vi "Serial_W_R with Files.vi"() -> ()   [LabVIEW 2022 SP3]
doc: "This example performs writes and reads on a serial port, as directed by the user. You can press the Write and Read buttons, and change the Read Count, while the example is running.\n\nThe parameters set for the serial port must match the parameters of the connected instrument or device. In this example, the Read Count parameter specifies the number of bytes that the serial port reads. If there were more bytes at the port than the specified number, those bytes would not be read. If there were less bytes at the port than the specified number, you would receive a timeout error.\n\nThis example expands upon the flow control options for XON and XOFF, allowing the user to choose those control characters. Also, the user can enable or disable a termination character. Some devices require a termination character in order to identify the end of command strings. Some devices send a termination character to signify the end of data to be read. This example shows how you can end the Read operation once a termination character is detected in the buffer and/or append a termination character at the end of the Write data."
uses:
  Applications/National Instruments/LabVIEW 2022 64-bit/examples/Instrument IO/Serial/support/Serial - Settings.ctl
  Applications/National Instruments/LabVIEW 2022 64-bit/examples/Instrument IO/Serial/support/Serial - ASCII Characters.ctl
  Applications/National Instruments/LabVIEW 2022 64-bit/examples/Instrument IO/Serial/support/Serial - XON-XOFF Characters.ctl
  Command_buttons.ctl
  <vilib>/Instr/_visa.llb/VISA Configure Serial Port (Instr).vi
  fg_enum.ctl
panel:
  in  "Stop Tx":bool
  in  "Temperature\nto set":dbl
  in  "Command Radio\nButtons":T1
  out "Response":string
  in  "Write":bool
  in  "Read":bool
  in  "VISA resource name":refnum<visa-resource-name>="COM1"
  # "------------------------\nPROGRAM EXECUTION   \n------------------------\n1. Connect PolyStat controller to PC via RS232 cable and choose corresponding port in 'VISA resource name'\n2. Set the time to poll which decides the time interval between each write-read pair or how often the command must be written and read\n3. Choose command to run by clicking the Radio buttons (can be changed during run). Refer the COMMANDS description for correct usage.\n4. Set the read and write buttons to ON for continuous polling mode\n5. Response can be observed on the given Response indicator\n6. Saved log PolyState_LabVIEW_log.txt can be found at LabVIEW default directory\n\nNOTE:\n> Only one command can be sent at a time\n> Program execution stops if controller response is negative\n> Program execution stops with error if no response is received from controller within 12 seconds after write\n> Time to poll cannot be changed during run, it is only read once at start"
  # "--------------\nCOMMANDS\n--------------\nP0 => Power off and standby\nP1 => Power on from standby\nF? => query fluid temperature\nS? => query current set temperature\nSn => set temperature to value n (change number between -40 to 105)\nValue of n should be given in 'Temperature to set' control\nUC => set unit to Celsius\nUF => set unit to Fahrenheit"
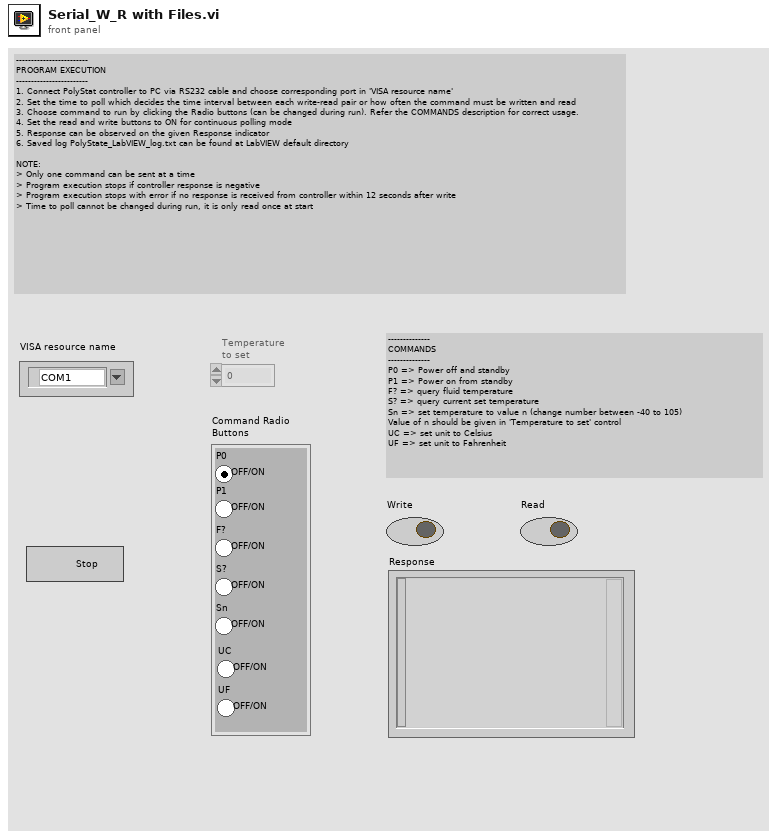
[diagram p1: front panel]
types:
  T1 = typedef "Command_buttons.ctl" = enum32{"P0", "P1", "F?", "S?", "Sn", "UC", "UF"}
  T2 = typedef "fg_enum.ctl" = enum16{"SET", "RESET TIME", "GET"}
  T3 = enum16{"open", "replace", "create", "open or create", "replace or create", "replace or create with confirmation"}
  T4 = typedef "Serial - XON-XOFF Characters.ctl" = cluster{"XON":T5, "XOFF":T5}
  T5 = typedef "Serial - ASCII Characters.ctl" = enum16{"NUL", "SOH", "STX", "ETX", "EOT", "ENQ", "ACK", "BEL", "BS", "HT", "LF", "VT", "FF", "CR", "SO", "SI", "DLE", "DC1", "DC2", "DC3", "DC4", "NAK", "SYN", "ETB", "CAN", "EM", "SUB", "ESC", "FS", "GS", "RS", "US", "SP", "!", "\"", "#", "$", "%", "&", "'", "(", ")", "*", "+", ",", "- (-)", ".", "/", "0", "1", "2", "3", "4", "5", "6", "7", "8", "9", ":", ";", "<", "=", ">", "?", "@", "A", "B", "C", "D", "E", "F", "G", "H", "I", "J", "K", "L", "M", "N", "O", "P", "Q", "R", "S", "T", "U", "V", "W", "X", "Y", "Z", "[", "\\", "]", "^", "_", "`", "a", "b", "c", "d", "e", "f", "g", "h", "i", "j", "k", "l", "m", "n", "o", "p", "q", "r", "s", "t", "u", "v", "w", "x", "y", "z", "{", "|", "}", "~"}
  T6 = typedef "Serial - Settings.ctl" = cluster{"baud rate":u32, "data bits":u16, "parity":enum16{"None", "Odd", "Even", "Mark", "Space"}, "stop bits":u16, "flow control":u16}
  T7 = enum8{"Enabled", "Disabled", "Disabled and Grayed Out"}
  T8 = typedef "Written_command.ctl" = string
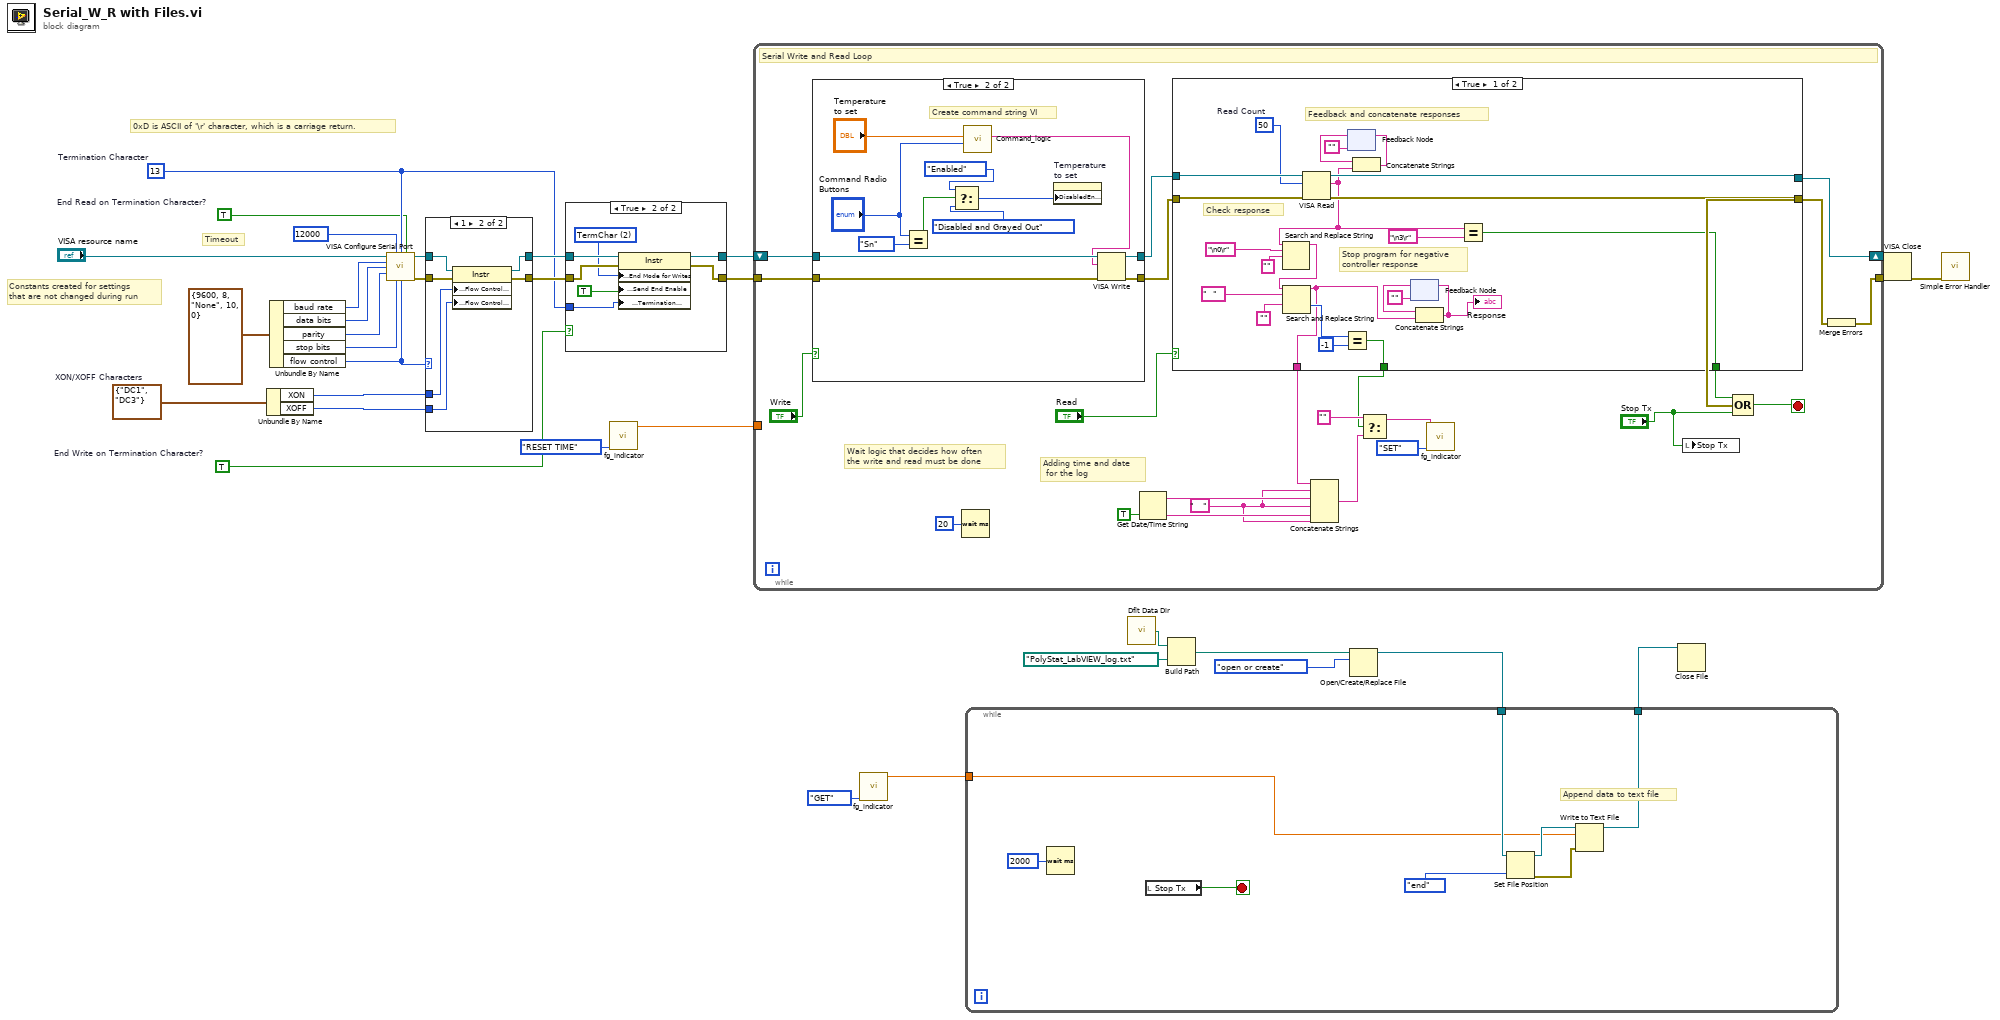
[diagram p0: block diagram]
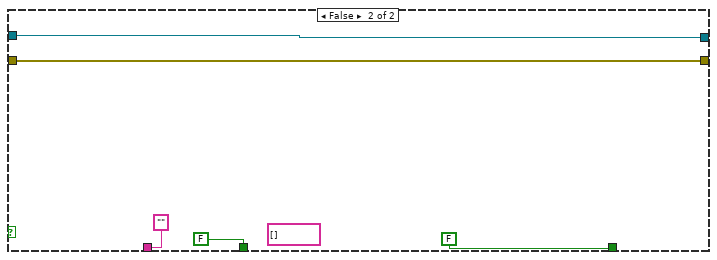
[diagram p5: hidden frame]
diagram:
  w12 = T4 {"XON"=enum."DC1", "XOFF"=enum."DC3"}  # XON/XOFF Characters
  w13 = TRUE  # End Write on Termination Character?
  w14 = TRUE  # End Read on Termination Character?
  w15 = u8 13  # Termination Character
  # "Constants created for settings\nthat are not changed during run"
  # "Timeout"
  # "0xD is ASCII of '\\r' character, which is a carriage return."
  n1 = Unbundle By Name(w12) -> ("XON"=w22:T5, "XOFF"=w21:T5)
  n2 = Unbundle By Name(T6 {"baud rate"=9600, "data bits"=8, "parity"=enum."None", "stop bits"=10, "flow control"=0} ("input cluster")) -> ("baud rate"=w27:u32, "data bits"=w28:u16, "parity"=w29:enum16{"None", "Odd", "Even", "Mark", "Space"}, "stop bits"=w30:u16, "flow control"=w23:u16)
  n3 = call-poly "VISA Configure Serial Port"("VISA resource name"="VISA resource name", "timeout (10sec)"=u32 12000, "termination char\n(0xA = '\\n' = LF)"=w15, "Enable Termination\nChar (T)"=w14, "baud rate (9600)"=w27, "data bits (8)"=w28, "parity (0:none)"=w29, "stop bits (10: 1 bit)"=w30, "flow control (0:none)"=w23) -> ("VISA resource name out"=w31:refnum<visa-resource-name>, "error out"=w32:errorcluster)  [unwired: 1 in, 4 out]
  n4 = case shown="1" w23 {
    tunnel: [w34 w41] -> w20
    tunnel: [w35 w40] -> w18
    tunnel: w32 -> [w34 w39]
    tunnel: w31 -> [w35 w38]
    tunnel: w22 -> [_ w37]
    tunnel: w21 -> [_ w36]
    frame Default {
    }
    frame 1 {
      n5 = property class="Instr"(reference=w38, error in=w39, "Serial Settings:Flow Control XON Character"=w37, "Serial Settings:Flow Control XOFF Character"=w36) -> (reference out=w40:refnum<visa-resource-name>, error out=w41:errorcluster)
    }
  }
  n6 = case shown="True" w13 {
    tunnel: w18 -> [w42 w50]
    tunnel: w20 -> [w43 w49]
    tunnel: [w42 w48] -> w17
    tunnel: [w43 w47] -> w19
    tunnel: w15 -> [_ w45]
    frame False {
    }
    frame True {
      w46 = u16 2 items=["None", "LastBit", "TermChar", "Break"] ("Serial Settings:Serial End Mode for Writes")
      n7 = property class="Instr"(reference=w50, error in=w49, "Serial Settings:End Mode for Writes"=w46, "Message Based Settings:Send End Enable"=TRUE, "Message Based Settings:Termination Character"=w45) -> (reference out=w48:refnum<visa-resource-name>, error out=w47:errorcluster)
    }
  }
  n8 = call "fg_indicator.vi"("Mode selector"=fg_enum."RESET TIME") -> ("Output"=w1:dbl)  [unwired: 8 in, 2 out]
  n9 = while {
    shift-right: [w73] -> w24
    shift-left: w17 -> [w72]
    tunnel: w19 -> [w71]
    tunnel: [w62] -> w25
    tunnel: w1 -> [_]
    stop <- w66 stop-if-true
    w56 = "   " ("string")
    # "Adding time and date\n for the log"
    # "Wait logic that decides how often\nthe write and read must be done"
    # "Serial Write and Read Loop"
    n10 = case shown="True" "Write" {
      tunnel: w72 -> [w75 w87]
      tunnel: w71 -> [w74 w86]
      tunnel: [w75 w85] -> w65
      tunnel: [w74 w84] -> w70
      frame False {
      }
      frame True {
        # "Create command string VI"
        n11 = Equal?(x="Command Radio\nButtons", y=Command_buttons."Sn") -> (x = y?=w77:bool)
        n12 = Select(t=T7."Enabled" ("Disabled"), s=w77, f=T7."Disabled and Grayed Out" ("Disabled")) -> (s? t:f=w76:T7)
        n13 = call "Command_logic.vi"("Command Radio Buttons"="Command Radio\nButtons", "Temperature\nto set"="Temperature\nto set") -> ("Written command"=w82:T8)  [unwired: 9 in]
        n14 = property on="Temperature\nto set" class="DigNum (strict)"("DisabledEnum"=w76) -> ()  [unwired: 2 in, 2 out]
        n15 = VISA Write(VISA resource name=w87, write buffer=w82, error in (no error)=w86) -> (VISA resource name out=w85:refnum<visa-resource-name>, error out=w84:errorcluster)  [unwired: 1 out]
      }
    }
    n16 = Wait (ms)(milliseconds to wait=u32 20) -> ()  [unwired: 1 out]
    n17 = Get Date/Time String(want seconds? (F)=TRUE) -> (date string=w58:string, time string=w57:string)  [unwired: 2 in]
    n18 = case shown="True" "Read" {
      tunnel: [w108 w115] -> w73
      tunnel: w65 -> [w110 w115]
      tunnel: [w107 w114] -> w63
      tunnel: w70 -> [w109 w114]
      tunnel: [w89 ""] -> w55
      tunnel: [w102 FALSE] -> w67
      tunnel: [w88 FALSE] -> w60
      frame True {
        w104 = u32 50  # Read Count
        # "Check response"
        # "Feedback and concatenate responses"
        # "Stop program for negative\ncontroller response"
        n19 = VISA Read(VISA resource name=w110, byte count=w104, error in (no error)=w109) -> (VISA resource name out=w108:refnum<visa-resource-name>, read buffer=w99:string, error out=w107:errorcluster)  [unwired: 1 out]
        n20 = Search and Replace String(input string=w99, search string="\n0\r" ("regular expression (\"\")"), replace string="" ("replace string (\"\")")) -> (result string=w95:string)  [unwired: 5 in, 3 out]
        n21 = Search and Replace String(input string=w95, search string="  " ("regular expression (\"\")"), replace string="" ("replace string (\"\")")) -> (result string=w89:string, offset past replacement=w94:i32)  [unwired: 5 in, 2 out]
        n22 = Equal?(x=w94, y=-1) -> (x = y?=w88:bool)
        n23 = feedback #1("") -> (w106:string)
        n24 = Concatenate Strings(w106, w99) -> (w98:string)
        n25 = feedback-in #1(w98) -> ()
        n26 = feedback #2("") -> (w91:string)
        n27 = Concatenate Strings(w91, w89) -> (w92:string)
        "Response" <- w92
        n28 = feedback-in #2(w92) -> ()
        n29 = Equal?(x=w99, y="\n3\r" ("regular expression (\"\")")) -> (x = y?=w102:bool)
      }
      frame False {
        (unwired) string[] []
      }
    }
    n30 = Concatenate Strings(w55, w56, w58, w56, w57, w56) -> (w54:string)
    n31 = Select(t="", s=w60, f=w54) -> (s? t:f=w53:string)
    n32 = call "fg_indicator.vi"("Mode selector"=fg_enum."SET", "Numeric"=w53) -> ()  [unwired: 7 in, 3 out]
    n33 = local write "Stop Tx"("Stop Tx") -> ()
    n34 = Compound Arithmetic op=OR(w67, w63, "Stop Tx") -> (w66:bool)
    n35 = Merge Errors(w63) -> (w62:errorcluster)
  }
  n36 = call "fg_indicator.vi"("Mode selector"=fg_enum."GET") -> ("Output"=w3:dbl)  [unwired: 8 in, 2 out]
  n37 = call <vilib>:"Dflt Data Dir.vi"() -> ("App:Default Data Directory"=w10:path)
  n38 = Build Path(base path=w10, name or relative path=path "PolyStat_LabVIEW_log.txt" ("default name")) -> (appended path=w7:path)
  n39 = Open/Create/Replace File(file path (use dialog)=w7, operation (0:open)=T3."open or create") -> (refnum out=w6:refnum<file>)  [unwired: 4 in, 2 out]
  n40 = while {
    tunnel: w6 -> [w119]
    tunnel: [w118] -> w5
    tunnel: w3 -> [w117]
    stop <- w116 stop-if-true
    # "Append data to text file"
    n41 = Wait (ms)(milliseconds to wait=u32 2000) -> ()  [unwired: 1 out]
    n42 = local read "Stop Tx"() -> (w116:bool)
    n43 = Set File Position(refnum=w119, from (0:start)=enum16{"start", "end", "current"}."end") -> (refnum out=w121:refnum<file>, error out=w120:errorcluster)  [unwired: 2 in]
    n44 = Write to Text File(file (use dialog)=w121, text=w117, error in=w120) -> (refnum out=w118:refnum<file>)  [unwired: 1 in, 2 out]
  }
  n45 = Close File(refnum=w5) -> ()  [unwired: 1 in, 2 out]
  n46 = VISA Close(VISA resource name=w24, error in (no error)=w25) -> (error out=w26:errorcluster)
  n47 = call <vilib>:"Simple Error Handler.vi"("error in (no error)"=w26) -> ()  [unwired: 1 in, 8 out]
